vi "Remove Duplicates from Array.vi"(11 "Array with Duplicates":u64[](array[numeric])) -> (3 "Cleaned Array":u64[](array[numeric]))   [LabVIEW 2013, in "Problem 3.lvlib"]
uses:
  Problem 3.lvlib
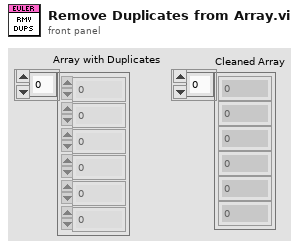
[diagram p1: front panel]
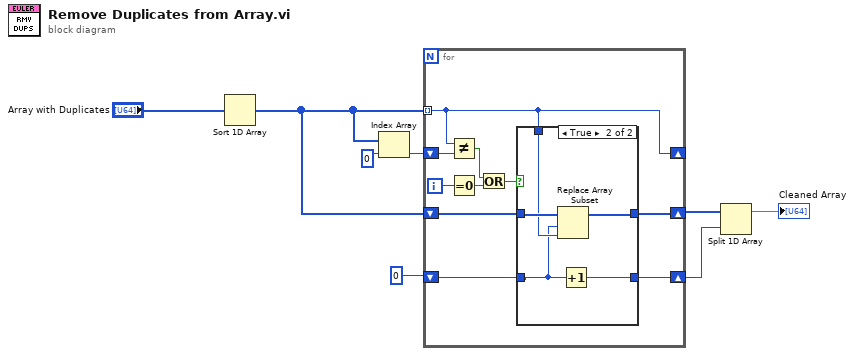
[diagram p0: block diagram]
diagram:
  n1 = Sort 1D Array(array="Array with Duplicates") -> (sorted array=w2:u64[])
  n2 = Index Array(array=w2, index=0) -> (element=w8:u64)
  n3 = for {
    tunnel: w2 -> [w11] mode=indexing
    shift-right: [w11] -> _
    shift-left: w8 -> [w15]
    shift-right: [w12] -> w5
    shift-left: w2 -> [w13]
    shift-right: [w9] -> w1
    shift-left: 0 ("index") -> [w10]
    i -> [w18]
    n4 = Not Equal?(x=w11, y=w15) -> (x != y?=w16:bool)
    n5 = Equal To 0?(x=w18) -> (x = 0?=w17:bool)
    n6 = Or(x=w16, y=w17) -> (x .or. y?=w14:bool)
    n7 = case shown="True" w14 {
      tunnel: w13 -> [w20 w25]
      tunnel: [w20 w21] -> w12
      tunnel: w11 -> [_ w24]
      tunnel: w10 -> [w19 w22]
      tunnel: [w19 w23] -> w9
      frame False {
      }
      frame True {
        n8 = Replace Array Subset(array=w25, new element=w24, index=w22) -> (w21:u64[])
        n9 = Increment(x=w22) -> (x+1=w23:i32)
      }
    }
  }
  n10 = Split 1D Array(array=w5, index=w1) -> (first subarray=→"Cleaned Array":u64[])  [unwired: 1 out]
